vi "update_dust_event_big.vi"(8 "error in (no error)":errorcluster, 11 "Cluster":T1 {"File Location" items=["Unknown"=-1, "Storage"=0, "Processing"=1, "Unmerged"=2]}) -> (0 "error out":errorcluster)   [LabVIEW 2013]
uses:
  <userlib>/Accelerator/User Interface/Controls/Post_Dust_Event.ctl
  <userlib>/Accelerator/User Interface/Controls/File_location.ctl
  <vilib>/addons/database/NI_Database_API.lvlib
panel:
  # "Dust Event"
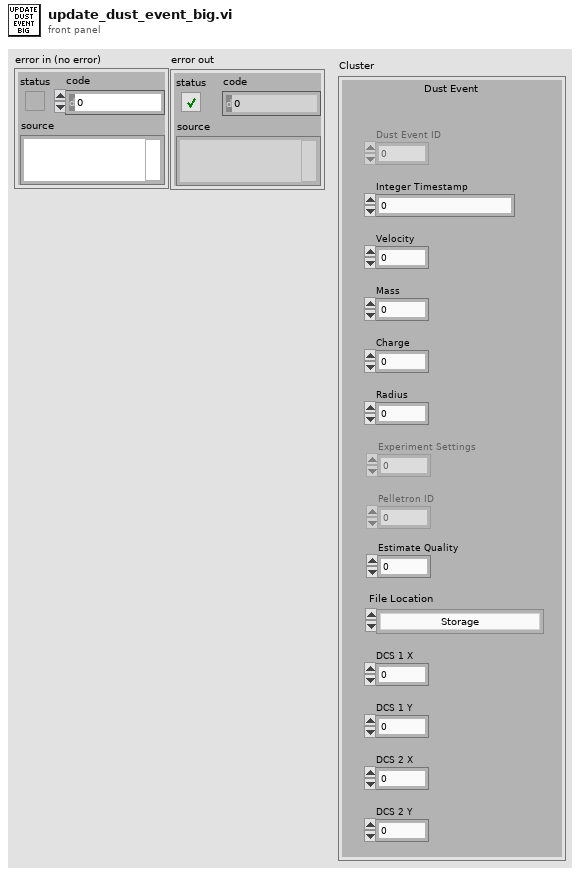
[diagram p1: front panel]
types:
  T1 = typedef "Post_Dust_Event.ctl" = cluster{"Dust Event ID":i64, "Integer Timestamp":i64, "Velocity":sgl, "Mass":sgl, "Charge":sgl, "Radius":sgl, "Experiment Settings":dbl, "Pelletron ID":i32, "Estimate Quality":sgl, "File Location":T2, "id_dust_info":dbl, "DCS 1 X":sgl, "DCS 1 Y":sgl, "DCS 2 X":sgl, "DCS 2 Y":sgl}
  T2 = typedef "File_location.ctl" = i8
  T3 = typedef "NI_Database_API.lvlib/Conn ObjectReference.ctl" = refnum<k1>
  T4 = cluster{"Velocity":sgl, "Mass":sgl, "Charge":sgl, "Radius":sgl, "Estimate Quality":sgl, "File Location":T2, "DCS 1 X":sgl, "DCS 1 Y":sgl, "DCS 2 X":sgl, "DCS 2 Y":sgl}
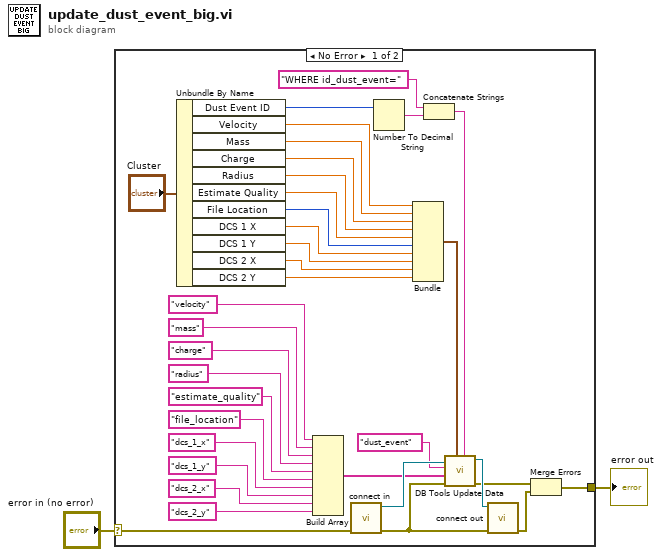
[diagram p0: block diagram]
diagram:
  n1 = case shown="No Error" "error in (no error)" {
    selector: "error in (no error)" -> [w36 w38]
    tunnel: [w33 w38] -> w1
    frame No Error {
      n2 = Unbundle By Name("Cluster") -> ("Dust Event ID"=w29:i64, "Velocity"=w14:sgl, "Mass"=w23:sgl, "Charge"=w22:sgl, "Radius"=w21:sgl, "Estimate Quality"=w20:sgl, "File Location"=w12:T2, "DCS 1 X"=w7:sgl, "DCS 1 Y"=w8:sgl, "DCS 2 X"=w9:sgl, "DCS 2 Y"=w10:sgl)
      n3 = Build Array("velocity" ("string"), "mass" ("string"), "charge" ("string"), "radius" ("string"), "estimate_quality" ("string"), "file_location" ("string"), "dcs_1_x" ("string"), "dcs_1_y" ("string"), "dcs_2_x" ("string"), "dcs_2_y" ("string")) -> (w24:string[])
      n4 = call <userlib>:"connect in.vi"("error in (no error)"=w36) -> ("error out"=w35:errorcluster, "Database Connection"=w37:T3)  [unwired: 7 in]
      n5 = Number To Decimal String(number=w29) -> (decimal integer string=w26:string)  [unwired: 1 in]
      n6 = Bundle("Velocity"=w14, "Mass"=w23, "Charge"=w22, "Radius"=w21, "Estimate Quality"=w20, "File Location"=w12, "DCS 1 X"=w7, "DCS 1 Y"=w8, "DCS 2 X"=w9, "DCS 2 Y"=w10) -> (w19:T4)  [unwired: 1 in]
      n7 = Concatenate Strings("WHERE id_dust_event=" ("condition"), w26) -> (w28:string)
      n8 = call <vilib>:"DB Tools Update Data.vi"("condition"=w28, "data"=w19, "error in (no error)"=w35, "columns"=w24, "table"="dust_event", "connection reference"=w37) -> ("error out"=w31:errorcluster, "connection reference out"=w32:T3)  [unwired: 4 in]
      n9 = call <userlib>:"connect out.vi"("error in (no error)"=w35, "connection reference"=w32) -> ("error out"=w34:errorcluster)  [unwired: 9 in]
      n10 = Merge Errors(w31, w34) -> (w33:errorcluster)
    }
    frame Error {
    }
  }
  "error out" <- w1
